vi "Inidicate The Last File of All Folder.vi"(11 "Root Folder":path) -> (3 "Last File Name":string)   [LabVIEW 2024]
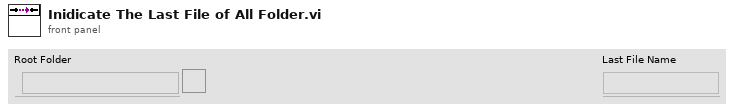
[diagram p1: front panel]
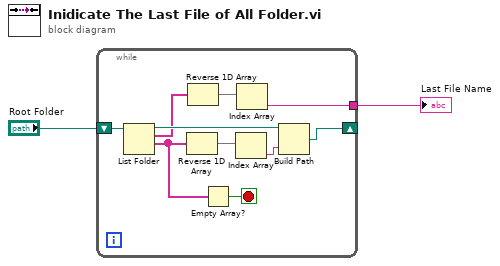
[diagram p0: block diagram]
diagram:
  n1 = while {
    shift-right: [w7] -> _
    shift-left: "Root Folder" -> [w12]
    tunnel: [w5] -> w1
    stop <- w3 stop-if-true
    n2 = List Folder(path=w12) -> (path out=w11:path, filenames=w4:string[], folder names=w10:string[])  [unwired: 3 in, 1 out]
    n3 = Reverse 1D Array(array=w10) -> (reversed array=w9:string[])
    n4 = Reverse 1D Array(array=w4) -> (reversed array=w6:string[])
    n5 = Empty Array?(array=w10) -> (empty?=w3:bool)
    n6 = Index Array(array=w9) -> (element=w8:string)  [unwired: 1 in]
    n7 = Index Array(array=w6) -> (element=w5:string)  [unwired: 1 in]
    n8 = Build Path(base path=w11, name or relative path=w8) -> (appended path=w7:path)
  }
  "Last File Name" <- w1
